vi "Resistance Measuring.vi"() -> ()   [LabVIEW 2022 SP3]
uses:
  2022 MPhys Project/Keithley 24XX Sweep and Acquire Measurements Folder/Keithley 24XX.lvlib
  2022 MPhys Project/Keithley 24XX Sweep and Acquire Measurements Folder/Public/Data/Read (Single Point).vi
panel:
  out "Voltage":sgl[](array[numeric])
  out "Resistance":sgl[](array[numeric])
  out "Current":sgl[](array[numeric])
  in  "Serial Configuration":T1={"Baud Rate"=9600, "Parity"=0, "Data Bits"=8, "Stop Bits"=10, "Flow Control"=0, "VISA resource name"=""} {"Flow Control" items=["None", "XON/XOFF", "RTS/CTS", "XON/XOFF & RTS/CTS", "DTR/DSR", "XON/XOFF & DTR/DSR"]; "Stop Bits" items=["1.0"=10, "1.5"=15, "2.0"=20]; "Data Bits" items=["7"=7, "8"=8]; "Parity" items=["None", "Odd", "Even", "Mark", "Space"]; "Baud Rate" items=["300"=300, "600"=600, "1200"=1200, "2400"=2400, "4800"=4800, "9600"=9600, "19200"=19200]}
  in  "Enable Resistance Auto Range (T:Enable)":bool=TRUE
  in  "Enable Current Auto Range (T:Enable)":bool=TRUE
  in  "Enable Voltage Auto Range (T:Enable)":bool=TRUE
  in  "Resistance Manual Range (1.0)":dbl=1.0
  in  "Current Manual Range (1.0)":dbl=1.0
  in  "Voltage Manual Range (1.0)":dbl=1.0
  in  "Output Level (0.1)":dbl=0.1
  in  "Compliance  Level (0.1)":dbl=0.1
  in  "Source Mode  (0: Voltage)":u16(ring) items=["Voltage", "Current"]
  in  "Number of measurement repeats":dbl
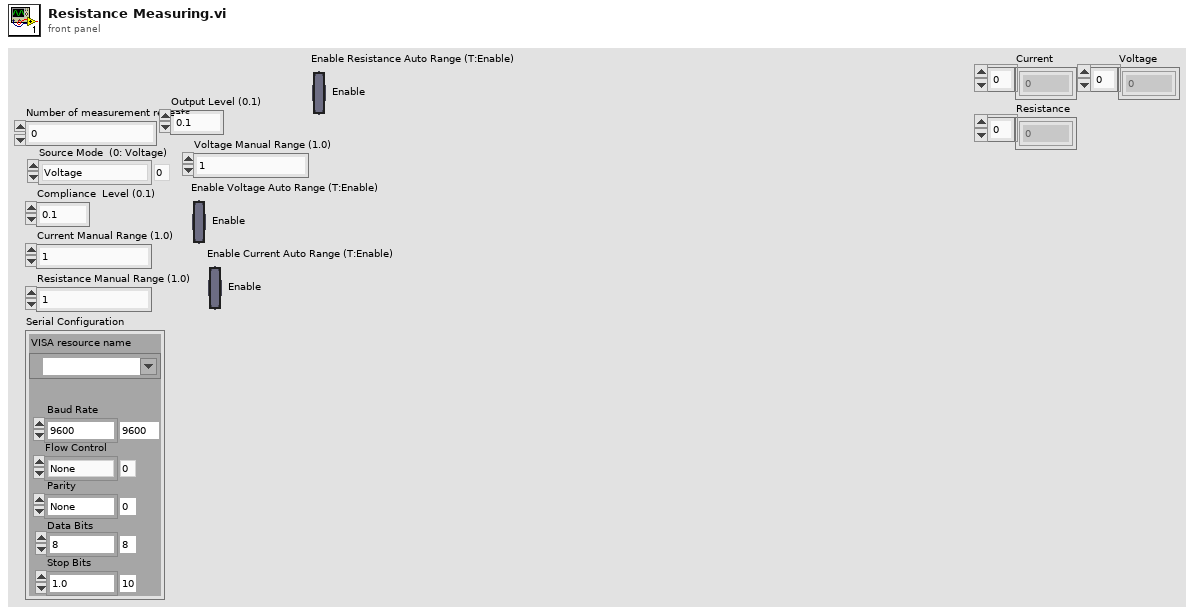
[diagram p1: front panel]
types:
  T1 = cluster{"Baud Rate":u32, "Parity":u16, "Data Bits":u16, "Stop Bits":u16, "Flow Control":u16, "VISA resource name":refnum<visa-resource-name>}
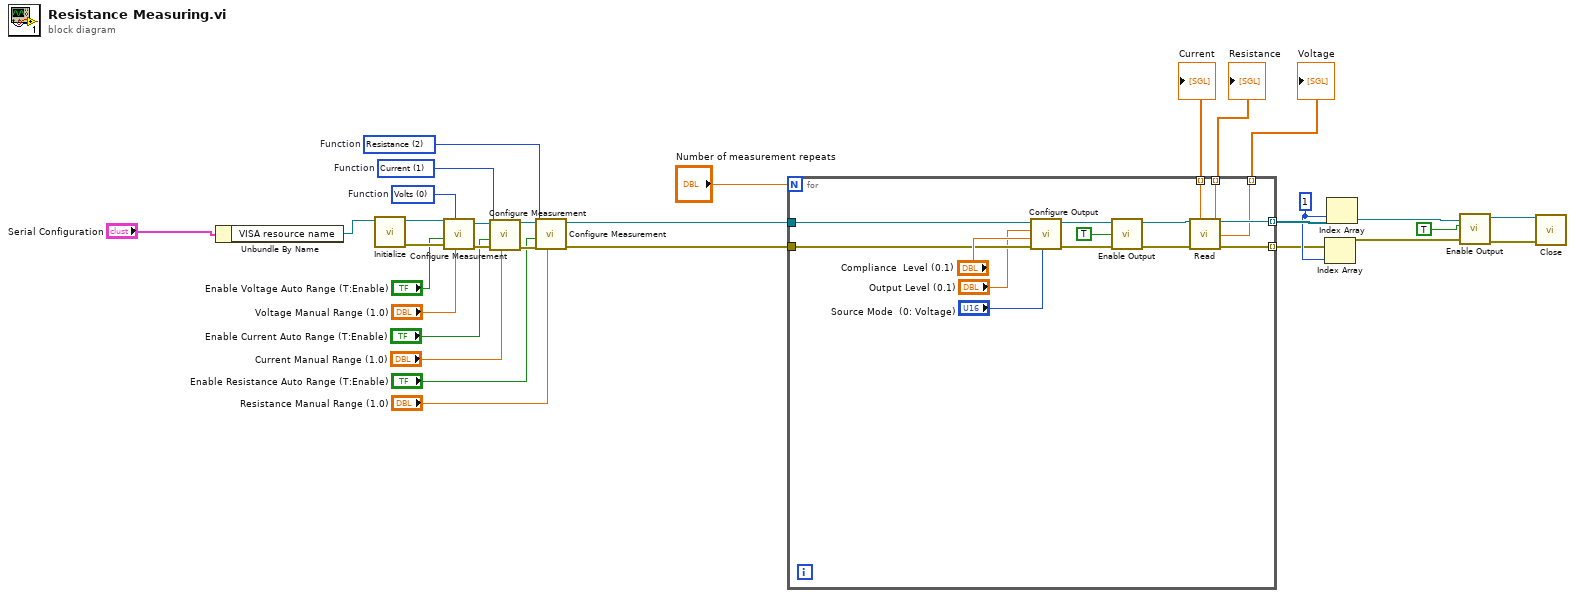
[diagram p0: block diagram]
diagram:
  w8 = 1
  w28 = u16 2 items=["Volts", "Current", "Resistance"]  # Function
  w29 = u16 1 items=["Volts", "Current", "Resistance"]  # Function
  w30 = u16 0 items=["Volts", "Current", "Resistance"]  # Function
  n1 = Unbundle By Name("Serial Configuration") -> ("VISA resource name"=w4:refnum<visa-resource-name>)
  n2 = call "Initialize.vi"("VISA resource name"=w4) -> ("error out"=w24:errorcluster, "VISA resource name out"=w27:refnum<visa-resource-name>)  [unwired: 9 in]
  n3 = call "Configure Measurement.vi"("Manual Range (1.0)"="Voltage Manual Range (1.0)", "error in (no error)"=w24, "Enable Auto Range (T:Enable)"="Enable Voltage Auto Range (T:Enable)", "Function (0: Volts)"=w30, "VISA resource name"=w27) -> ("error out"=w23:errorcluster, "VISA resource name out"=w26:refnum<visa-resource-name>)  [unwired: 5 in]
  n4 = call "Configure Measurement.vi"("Manual Range (1.0)"="Current Manual Range (1.0)", "error in (no error)"=w23, "Enable Auto Range (T:Enable)"="Enable Current Auto Range (T:Enable)", "Function (0: Volts)"=w29, "VISA resource name"=w26) -> ("error out"=w22:errorcluster, "VISA resource name out"=w25:refnum<visa-resource-name>)  [unwired: 5 in]
  n5 = call "Configure Measurement.vi"("Manual Range (1.0)"="Resistance Manual Range (1.0)", "error in (no error)"=w22, "Enable Auto Range (T:Enable)"="Enable Resistance Auto Range (T:Enable)", "Function (0: Volts)"=w28, "VISA resource name"=w25) -> ("error out"=w20:errorcluster, "VISA resource name out"=w21:refnum<visa-resource-name>)  [unwired: 5 in]
  n6 = for {
    N: "Number of measurement repeats" -> [_]
    tunnel: w21 -> [w41]
    tunnel: w20 -> [w40]
    tunnel: [w36] -> w7 mode=indexing
    tunnel: [w35] -> w10 mode=indexing
    tunnel: [w34] -> w3 mode=indexing
    tunnel: [w33] -> w2 mode=indexing
    tunnel: [w32] -> w1 mode=indexing
    n7 = call "Configure Output.vi"("Source Mode  (0: Voltage)"="Source Mode  (0: Voltage)", "error in (no error)"=w40, "Compliance  Level (0.1)"="Compliance  Level (0.1)", "Output Level (0)"="Output Level (0.1)", "VISA resource name"=w41) -> ("error out"=w37:errorcluster, "VISA resource name out"=w38:refnum<visa-resource-name>)  [unwired: 5 in]
    n8 = call "Enable Output.vi"("error in (no error)"=w37, "Enable Output (T: Enable)"=TRUE, "VISA resource name"=w38) -> ("error out"=w42:errorcluster, "VISA resource name out"=w43:refnum<visa-resource-name>)  [unwired: 7 in]
    n9 = call-poly "Read.vi"("VISA resource name"=w43, "error in (no error)"=w42) -> ("Voltage"=w32:sgl, "VISA resource name out"=w35:refnum<visa-resource-name>, "Current"=w34:sgl, "Resistance"=w33:sgl, "error out"=w36:errorcluster)  [unwired: 7 in, 2 out]
  }
  "Current" <- w3
  "Resistance" <- w2
  "Voltage" <- w1
  n10 = Index Array(array=w7, index=w8) -> (element=w6:errorcluster)
  n11 = Index Array(array=w10, index=w8) -> (element=w9:refnum<visa-resource-name>)
  n12 = call "Enable Output.vi"("error in (no error)"=w6, "Enable Output (T: Enable)"=TRUE, "VISA resource name"=w9) -> ("error out"=w12:errorcluster, "VISA resource name out"=w13:refnum<visa-resource-name>)  [unwired: 7 in]
  n13 = call "Close.vi"("error in (no error)"=w12, "VISA resource name"=w13) -> ()  [unwired: 9 in, 1 out]
